vi "FPGA.vi"() -> ()   [LabVIEW 2015]
uses:
  <vilib>/rvi/Emulation/niFpgaGetClockAttributes.vi
  <vilib>/rvi/Emulation/niFpgaSctlEmulationGetInTimedLoop.vi
  <vilib>/rvi/Emulation/niFpgaEmulationReportErrorSimple.vi
  <vilib>/rvi/eio/common/nirviEmuTemplateMethod_errors.vi
  <vilib>/rvi/Emulation/niFpgaCriticalErrorInLSC.vi
  <vilib>/eio/EIONode/EIONode.xnode
  <vilib>/rvi/FXPMathLib/FxpMul/XNode/nifxpmath_Multiplier.xnode
  <vilib>/rvi/FXPMathLib/sim/FxpSim.dll
panel:
  out "u(k)":fxp<+,20,0>
  out "vB(k)_op":fxp<+,28,8>
  out "T":u32
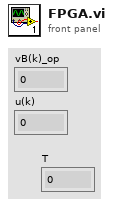
[diagram p1: front panel]
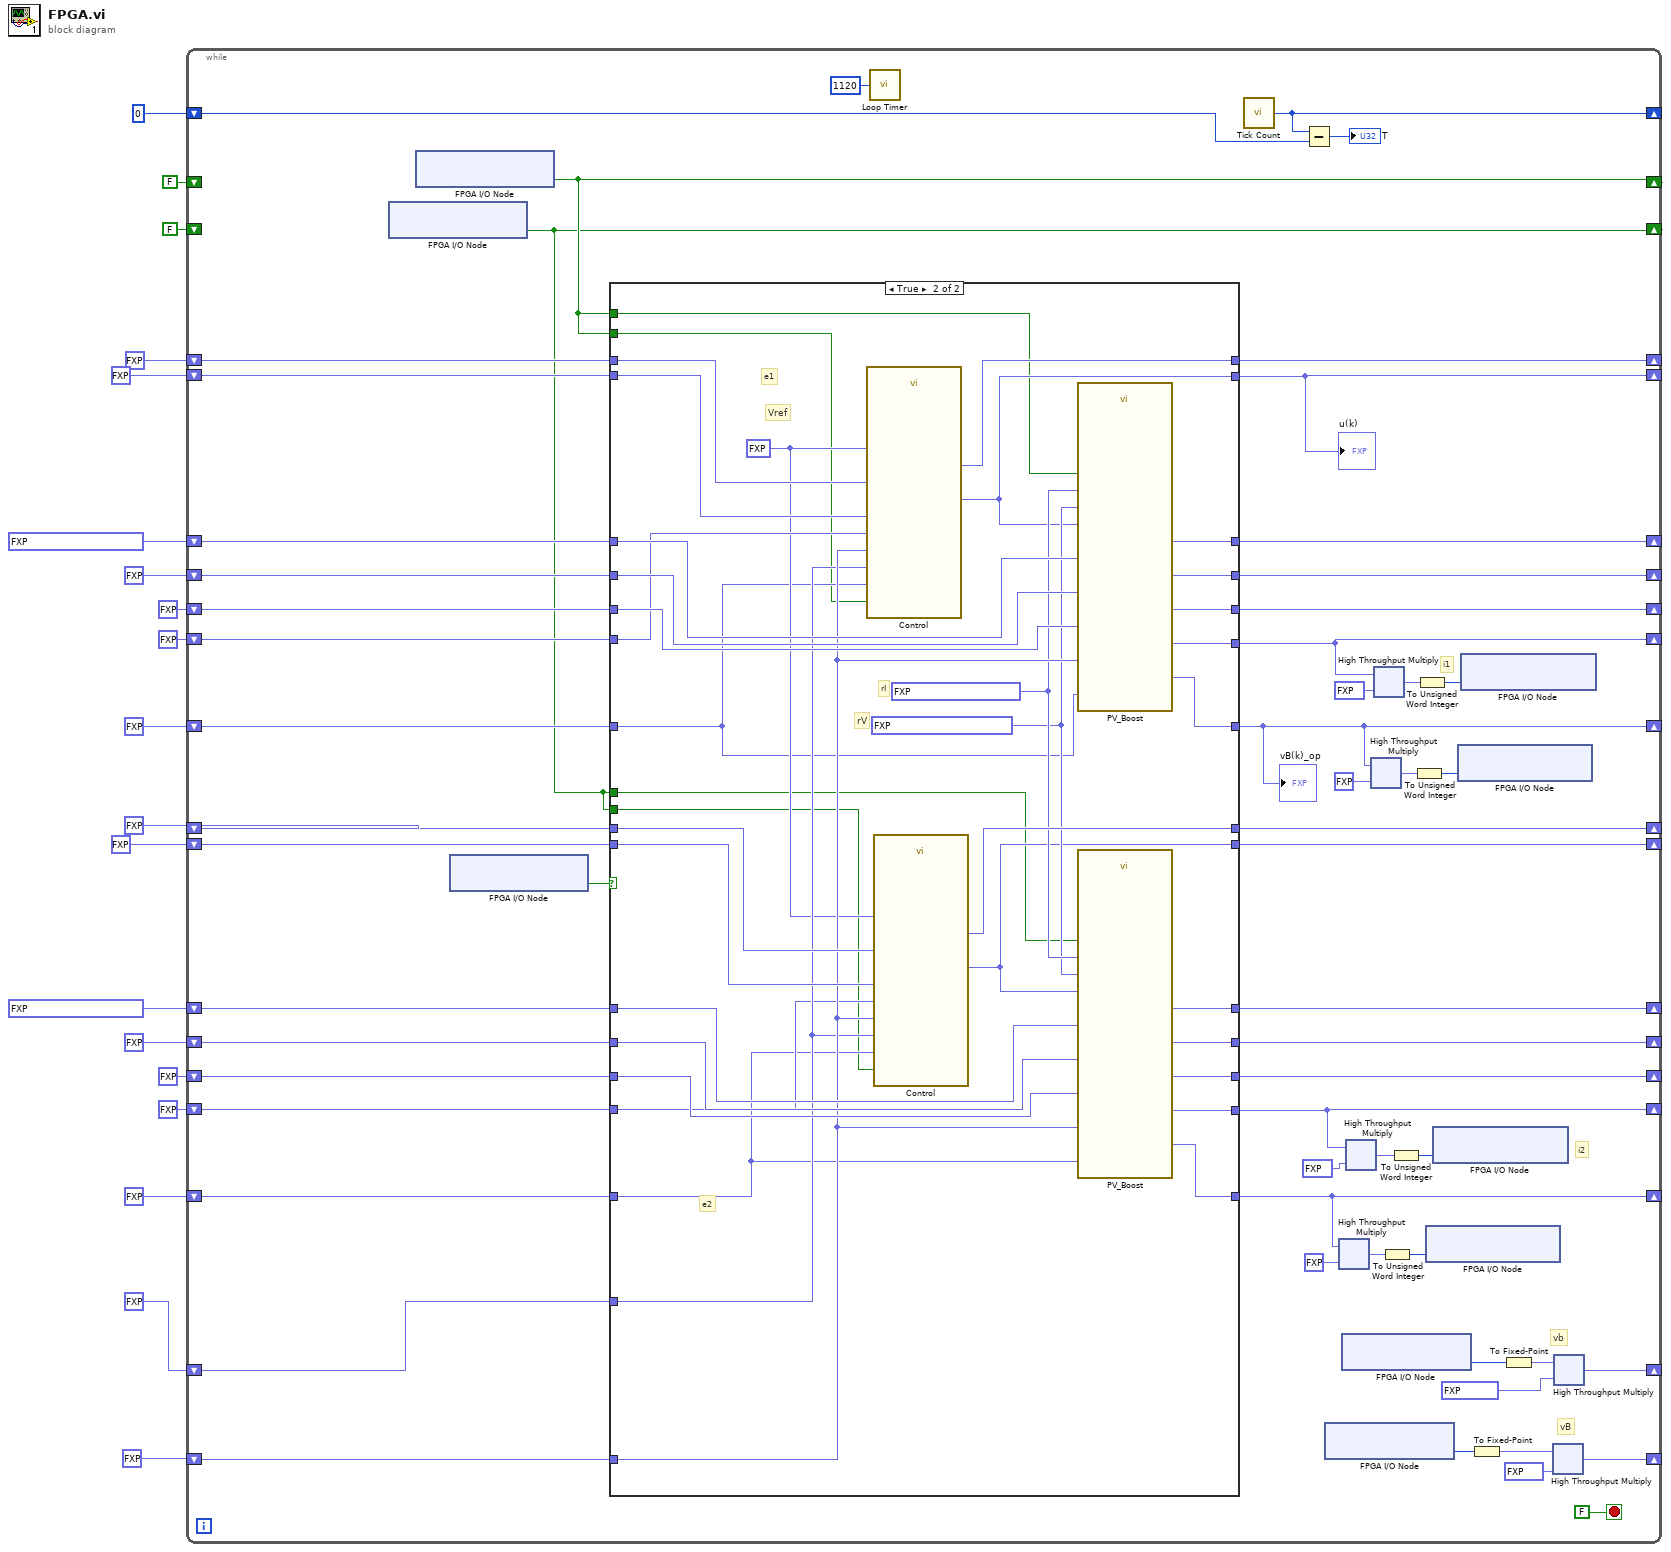
[diagram p0: block diagram]
diagram:
  n1 = while {
    shift-right: [w36] -> _
    shift-left: fxp<+,28,8> 0.0 ("vB") -> [w58]
    shift-right: [w39] -> _
    shift-left: fxp<+,24,4> 0.0 ("x*y") -> [w57]
    shift-right: [w44] -> _
    shift-left: fxp<+/-,25,5> 0.0 ("Io") -> [w46]
    shift-right: [w45] -> _
    shift-left: fxp<+/-,25,5> 0.0 ("Io") -> [w47]
    shift-right: [w76] -> _
    shift-left: fxp<+/-,29,9> 0.0 ("e(k)") -> [w75]
    shift-right: [w29] -> _
    shift-left: fxp<+,20,0> 0.0 ("u(k)") -> [w74]
    shift-right: [w71] -> _
    shift-left: fxp<+/-,27,7> 0.0 ("i_L_P(k)") -> [w68]
    shift-right: [w72] -> _
    shift-left: fxp<+,24,4> 0.0 ("i_pv(k)") -> [w69]
    shift-right: [w73] -> _
    shift-left: fxp<+,26,6> 37.85000038146973 ("v_pv(k)") -> [w70]
    shift-right: [w67] -> _
    shift-left: fxp<+/-,29,9> 0.0 ("e(k)") -> [w66]
    shift-right: [w28] -> _
    shift-left: fxp<+,20,0> 0.0 ("u(k)") -> [w65]
    shift-right: [w64] -> _
    shift-left: fxp<+,26,6> 37.85000038146973 ("v_pv(k)") -> [w61]
    shift-right: [w63] -> _
    shift-left: fxp<+,24,4> 0.0 ("i_pv(k)") -> [w60]
    shift-right: [w62] -> _
    shift-left: fxp<+/-,27,7> 0.0 ("i_L_P(k)") -> [w59]
    shift-right: [w50] -> _
    shift-left: u32 0 ("Tick Count(Ticks)") -> [w49]
    shift-right: [w25] -> _
    shift-left: fxp<+,28,8> 0.0 ("vB(k)_op") -> [w27]
    shift-right: [w24] -> _
    shift-left: fxp<+,28,8> 0.0 ("vB(k)_op") -> [w26]
    shift-right: [w21] -> _
    shift-left: FALSE ("ConnectorA/DIO0") -> [_]
    shift-right: [w20] -> _
    shift-left: FALSE ("ConnectorA/DIO1") -> [_]
    stop <- FALSE stop-if-true
    # "i2"
    # "i1"
    # "vB"
    # "vb"
    n2 = xnode "FPGA I/O Node"() -> ("ConnectorA/DIO1"=w20:bool)  [unwired: 1 in, 1 out]
    n3 = xnode "FPGA I/O Node"() -> ("ConnectorA/DIO0"=w21:bool)  [unwired: 1 in, 1 out]
    n4 = xnode "FPGA I/O Node"() -> ("ConnectorA/DIO2"=w22:bool)  [unwired: 1 in, 1 out]
    n5 = case shown="True" w22 {
      tunnel: [w91 w128] -> w76
      tunnel: w75 -> [w91 w127]
      tunnel: w74 -> [w90 w126]
      tunnel: [w89 w125] -> w73
      tunnel: [w88 w124] -> w72
      tunnel: [w87 w123] -> w71
      tunnel: w70 -> [w89 w122]
      tunnel: w69 -> [w88 w121]
      tunnel: w68 -> [w87 w120]
      tunnel: [w84 w119] -> w67
      tunnel: w66 -> [w84 w118]
      tunnel: w65 -> [w83 w117]
      tunnel: [w82 w116] -> w64
      tunnel: [w81 w115] -> w63
      tunnel: [w80 w114] -> w62
      tunnel: w61 -> [w82 w113]
      tunnel: w60 -> [w81 w112]
      tunnel: w59 -> [w80 w111]
      tunnel: w58 -> [_ w110]
      tunnel: w57 -> [_ w109]
      tunnel: w47 -> [w86 w108]
      tunnel: w46 -> [w79 w107]
      tunnel: [w86 w106] -> w45
      tunnel: [w79 w105] -> w44
      tunnel: [w85 w101] -> w25
      tunnel: [w78 w100] -> w24
      tunnel: [w90 w99] -> w29
      tunnel: [w83 w98] -> w28
      tunnel: w27 -> [w85 w97]
      tunnel: w21 -> [_ w96]
      tunnel: w26 -> [w78 w95]
      tunnel: w20 -> [_ w92]
      tunnel: w21 -> [_ w94]
      tunnel: w20 -> [_ w93]
      frame False {
      }
      frame True {
        w102 = fxp<+,25,5> 27.02774143218994 ("r_V1")
        w103 = fxp<+,20,0> 0.0001316070556640625 ("r_I1")
        w104 = fxp<+,28,8> 190.0 ("v_ref")
        # "rV"
        # "rI"
        # "e2"
        # "e1"
        # "Vref"
        n6 = call "Control.vi"("vB"=w110, "vB_o"=w97, "Vb"=w109, "e(k-1)"=w127, "s_c"=w94, "Io"=w108, "u(k-1)"=w126, "v_ref"=w104) -> ("u(k)"=w99:fxp<+,20,0>, "e(k)"=w128:fxp<+/-,29,9>)  [unwired: 2 in]
        n7 = call "Control.vi"("vB"=w110, "vB_o"=w95, "Vb"=w109, "e(k-1)"=w118, "s_c"=w93, "Io"=w107, "u(k-1)"=w117, "v_ref"=w104) -> ("u(k)"=w98:fxp<+,20,0>, "e(k)"=w119:fxp<+/-,29,9>)  [unwired: 2 in]
        n8 = call "PV_Boost.vi"("i_pv(k-1)"=w121, "D"=w99, "r_V(G)"=w102, "v_pv(k-1)"=w122, "vB(k-1)_op"=w97, "i_L_P(k-1)"=w120, "e"=w96, "vB(k-1)"=w110, "r_I(G)"=w103) -> ("i_pv(k)"=w124:fxp<+,24,4>, "v_pv(k)"=w125:fxp<+,26,6>, "vB(k)_op"=w101:fxp<+,28,8>, "i_L_P(k)"=w123:fxp<+/-,27,7>, "Io"=w106:fxp<+/-,25,5>)  [unwired: 2 in]
        n9 = call "PV_Boost.vi"("i_pv(k-1)"=w112, "D"=w98, "r_V(G)"=w102, "v_pv(k-1)"=w113, "vB(k-1)_op"=w95, "i_L_P(k-1)"=w111, "e"=w92, "vB(k-1)"=w110, "r_I(G)"=w103) -> ("i_pv(k)"=w115:fxp<+,24,4>, "v_pv(k)"=w116:fxp<+,26,6>, "vB(k)_op"=w100:fxp<+,28,8>, "i_L_P(k)"=w114:fxp<+/-,27,7>, "Io"=w105:fxp<+/-,25,5>)  [unwired: 2 in]
      }
    }
    "vB(k)_op" <- w25
    "u(k)" <- w29
    n10 = call "Loop Timer"("Count(Ticks)"=u32 1120) -> ()  [unwired: 1 out]
    n11 = call "Tick Count"() -> ("Tick Count(Ticks)"=w50:u32)
    n12 = Subtract(x=w50, y=w49) -> (x-y=→"T":u32)
    n13 = xnode "FPGA I/O Node"() -> ("ConnectorA/AI1"=w42:u16)  [unwired: 1 in, 1 out]
    n14 = xnode ("High Throughput Multiply")("x"=w24, "y"=fxp<+,5,5> 16.0) -> ("x*y"=w32:fxp<+,16,16>)
    n15 = xnode "FPGA I/O Node"() -> ("ConnectorA/AI0"=w43:u16)  [unwired: 1 in, 1 out]
    n16 = xnode ("High Throughput Multiply")("x"=w44, "y"=fxp<+,11,11> 1024.0) -> ("x*y"=w53:fxp<+,16,16>)
    n17 = xnode ("High Throughput Multiply")("x"=w25, "y"=fxp<+,5,5> 16.0) -> ("x*y"=w33:fxp<+,16,16>)
    n18 = xnode ("High Throughput Multiply")("x"=w45, "y"=fxp<+,11,11> 1024.0) -> ("x*y"=w56:fxp<+,16,16>)
    n19 = To Unsigned Word Integer(number=w32) -> (unsigned 16bit integer=w31:u16)
    n20 = To Unsigned Word Integer(number=w53) -> (unsigned 16bit integer=w52:u16)
    n21 = To Unsigned Word Integer(number=w33) -> (unsigned 16bit integer=w34:u16)
    n22 = To Unsigned Word Integer(number=w56) -> (unsigned 16bit integer=w55:u16)
    n23 = xnode "FPGA I/O Node"("ConnectorB/AO1"=w31) -> ()  [unwired: 1 in, 1 out]
    n24 = xnode "FPGA I/O Node"("ConnectorA/AO1"=w52) -> ()  [unwired: 1 in, 1 out]
    n25 = xnode "FPGA I/O Node"("ConnectorB/AO0"=w34) -> ()  [unwired: 1 in, 1 out]
    n26 = xnode "FPGA I/O Node"("ConnectorA/AO0"=w55) -> ()  [unwired: 1 in, 1 out]
    n27 = To Fixed-Point(number=w42) -> (fixed-point=w37:fxp<+,16,16>)  [unwired: 1 in]
    n28 = To Fixed-Point(number=w43) -> (fixed-point=w41:fxp<+,16,16>)  [unwired: 1 in]
    n29 = xnode ("High Throughput Multiply")("x"=w37, "y"=fxp<+,4,0> 0.0625) -> ("x*y"=w36:fxp<+,28,8>)
    n30 = xnode ("High Throughput Multiply")("x"=w41, "y"=fxp<+,7,0> 0.0078125) -> ("x*y"=w39:fxp<+,24,4>)
  }
